vi "TranslateStrings.vi"(8 "error in (no error)":errorcluster, 11 "String Array":string[](array[string])) -> (0 "error out":errorcluster, 3 "Translated string array":string[](array[string]))   [LabVIEW 2011]
uses:
  Dictionnary/EnumCommandDictionnaire.ctl
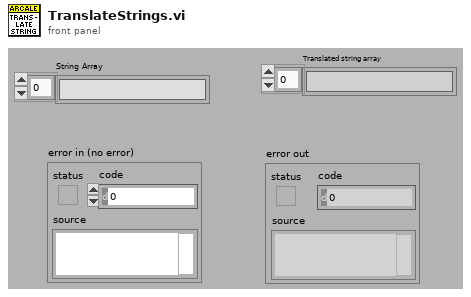
[diagram p1: front panel]
types:
  T1 = typedef "EnumCommandDictionnaire.ctl" = enum16{"Load", "Translate", "Save", "GetDico", "Set : A traduire = Vrai", "Set : A Traduire = Faux", "SetDico"}
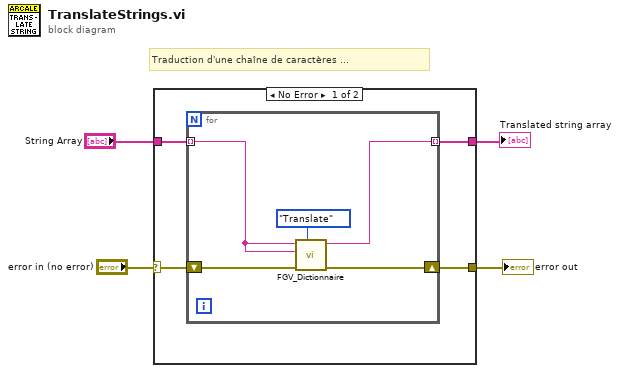
[diagram p0: block diagram]
diagram:
  # "Traduction d'une chaîne de caractères ..."
  n1 = case shown="No Error" "error in (no error)" {
    selector: "error in (no error)" -> [w5 w15]
    tunnel: [w8 w15] -> w3
    tunnel: "String Array" -> [w7 w14]
    tunnel: [w6 w14] -> w1
    frame No Error {
      n2 = for {
        shift-right: [w11] -> w8
        shift-left: w5 -> [w12]
        tunnel: w7 -> [w10] mode=indexing
        tunnel: [w9] -> w6 mode=indexing
        n3 = call "FGV_Dictionnaire.vi"("Command"=EnumCommandDictionnaire."Translate", "error in (no error)"=w12, "Chaîne"=w10, "Clé"=w10) -> ("error out"=w11:errorcluster, "Traduction"=w9:string)  [unwired: 5 in, 1 out]
      }
    }
    frame Error {
    }
  }
  "error out" <- w3
  "Translated string array" <- w1
